vi "InTurnBoatMode.vi"() -> ()   [LabVIEW 2012]
doc: "Write an algorithm that returns 'true' when the desired heading and the robot heading are more than 30 (that's arbitrary for now) degrees apart, except that the algorithm should return false if going from the robot heading to the desired heading involves crossing the wind, upwind or downwind.\n\nSo, to clarify:\nRH and DH less than 30 degrees apart: False\nRH and DH more than 30 degrees apart, but going from RH to DH involves crossing the wind: False\nRH and DH more than 30 degrees apart: True\n\nEric Schneider, Jan. 2014"
uses:
  Utilities/Math/Angles/Angle/Angle.lvclass
panel:
  in  "RobotHeading (0-360)":dbl(knob)
  out "InTurnBoatMode?":bool
  in  "DifferenceCutoff":i32=30
  in  "AbsoluteWind (0-360)":dbl
  in  "stop 3":bool
  in  "DesiredHeading (0-360)":dbl(knob)
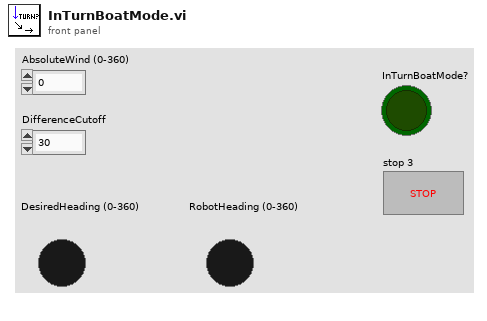
[diagram p1: front panel]
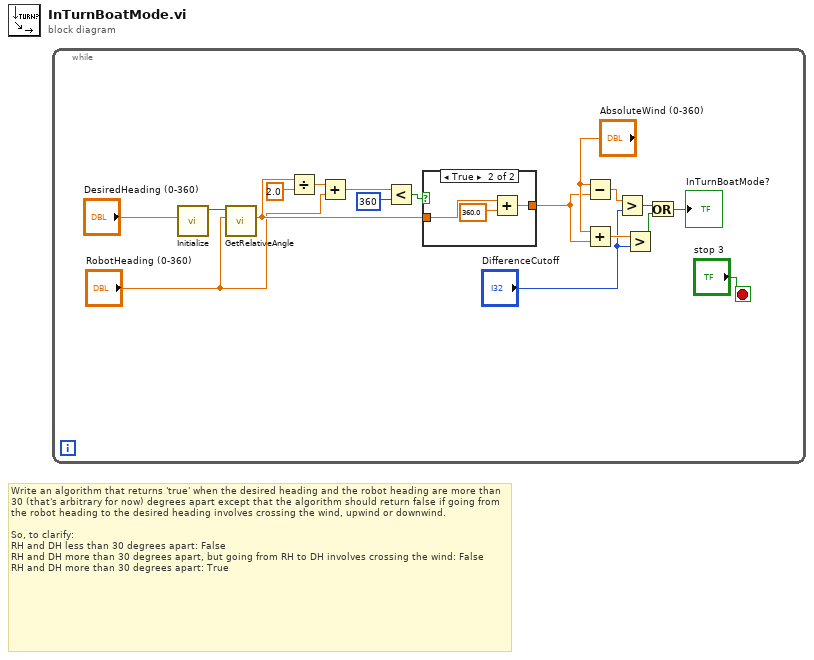
[diagram p0: block diagram]
diagram:
  # "Write an algorithm that returns 'true' when the desired heading and the robot heading are more than 30 (that's arbitrary for now) degrees apart except that the algorithm should return false if going from the robot heading to the desired heading involves crossing the wind, upwind or downwind.\n\nSo, to clarify:\nRH and DH less than 30 degrees apart: False\nRH and DH more than 30 degrees apart, but going from RH to DH involves crossing the wind: False\nRH and DH more than 30 degrees apart: True"
  n1 = while {
    stop <- "stop 3" stop-if-true
    n2 = call "Initialize.vi"("Input Angle (Deg.)"="DesiredHeading (0-360)") -> ("Angle out"=w17:refnum<class "Angle.lvclass">)  [unwired: 9 in, 1 out]
    n3 = call "GetRelativeAngle.vi"("Boat Heading (Deg.)"="RobotHeading (0-360)", "Angle in"=w17) -> ("Relative Angle"=w13:dbl)  [unwired: 8 in, 1 out]
    n4 = Divide(x=w13, y=2.0) -> (x/y=w11:dbl)
    n5 = Add(x=w11, y="RobotHeading (0-360)") -> (x+y=w9:dbl)
    n6 = Less?(x=w9, y=360) -> (x < y?=w15:bool)
    n7 = case shown="True" w15 {
      tunnel: w13 -> [w19 w22]
      tunnel: [w19 w20] -> w1
      frame False {
      }
      frame True {
        n8 = Add(x=w22, y=360.0) -> (x+y=w20:dbl)
      }
    }
    n9 = Subtract(x="AbsoluteWind (0-360)", y=w1) -> (x-y=w5:dbl)
    n10 = Add(x="AbsoluteWind (0-360)", y=w1) -> (x+y=w8:dbl)
    n11 = Greater?(x=w5, y="DifferenceCutoff") -> (0:w4:bool)
    n12 = Greater?(x=w8, y="DifferenceCutoff") -> (0:w7:bool)
    n13 = Or(x=w4, y=w7) -> (x .or. y?=→"InTurnBoatMode?":bool)
  }
